vi "Resize.vi"(8 "error in (no error)":errorcluster, 10 "Width":i32, 11 "TermLine in":refnum<class "TermLine.lvclass">) -> (0 "error out":errorcluster, 3 "TermLine out":refnum<class "TermLine.lvclass">)   [LabVIEW 2020, in "Terminal.lvlib" / "TermLine.lvclass"]
uses:
  TermLine.lvclass
  TermLine.lvclass/TermLine.ctl
  Term Char.ctl
  Terminal.lvlib
  Text Attributes.ctl
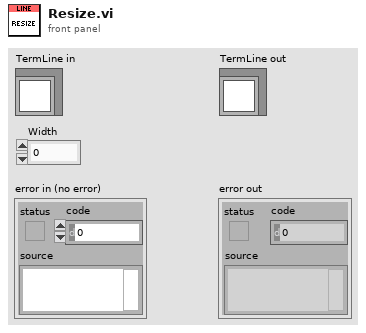
[diagram p1: front panel]
types:
  T1 = typedef "Terminal.lvlib/Term Char.ctl" = cluster{"Char":string, "Attributes":T2}
  T2 = typedef "Terminal.lvlib/Text Attributes.ctl" = cluster{"FG":u32, "BG":u32, "Bold":bool, "Italic":bool, "Underline":bool, "Strike":bool, "Inverse":bool}
  T3 = typedef "Terminal.lvlib/TermLine.lvclass/Ref Data.ctl" = cluster{"Chars":T1[], "Width":i32}
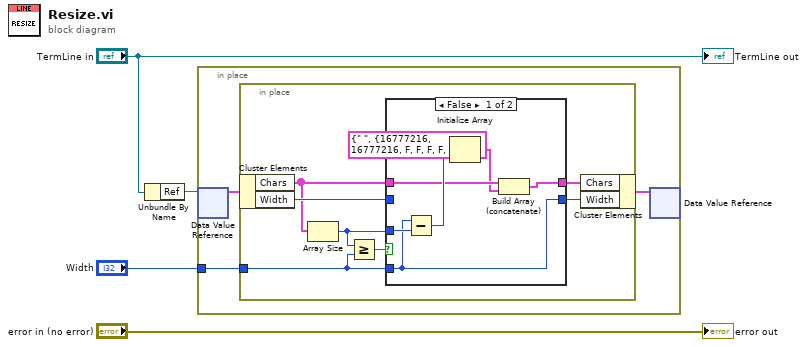
[diagram p0: block diagram]
diagram:
  n1 = Unbundle By Name("TermLine in") -> ("Ref"=w3:refnum<data-value>)
  n2 = in-place {
    in-place-border: "Width" -> [w5]
    n3 = in-place-dvr #1(w3) -> (w7:T3)  [unwired: 1 out]
    n4 = in-place {
      in-place-border: w5 -> [w12]
      n5 = in-place-cluster #2(w7) -> ("Chars"=w10:T1[], "Width"=w11:i32)
      n6 = Array Size(array=w10) -> (size(s)=w13:i32)
      n7 = Greater Or Equal?(x=w13, y=w12) -> (x >= y?=w14:bool)
      n8 = case shown="False" w14 {
        tunnel: w13 -> [w21 _]
        tunnel: w12 -> [w18 w22]
        tunnel: w11 -> [_ _]
        tunnel: w10 -> [w17 w23]
        tunnel: [w15 w23] -> w9
        tunnel: [w18 w22] -> w8
        frame False {
          n9 = Subtract(x=w18, y=w21) -> (x-y=w19:i32)
          n10 = Initialize Array(T1 {"Char"=" ", "Attributes"={"FG"=16777216, "BG"=16777216, "Bold"=FALSE, "Italic"=FALSE, "Underline"=FALSE, "Strike"=FALSE, "Inverse"=FALSE}} ("Term Char"), w19) -> (w16:T1[])
          n11 = Build Array (concatenate)(w17, w16) -> (w15:T1[])
        }
        frame True {
          # "Already have at least enough width"
        }
      }
      n12 = in-place-cluster #2("Chars"=w9, "Width"=w8) -> (w6:T3)
    }
    n13 = in-place-dvr #1(w6) -> ()  [unwired: 2 out]
  }
  "error out" <- "error in (no error)"
  "TermLine out" <- "TermLine in"
